vi "_047.vi"() -> ()   [LabVIEW 2024]
panel:
  out "appended array":dbl[](array[numeric])
  out "initialized array 2":dbl[][](array[numeric])
  out "initialized array":dbl[](array[numeric])
  out "Array 4":i32[][](array[numeric])
  out "Array 3":i32[](array[numeric])
  in  "Array":dbl[](array[numeric])
  in  "Array":dbl[](array[numeric])
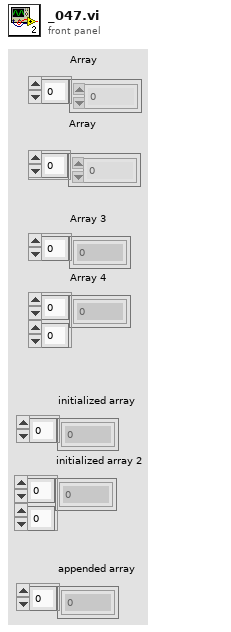
[diagram p1: front panel]
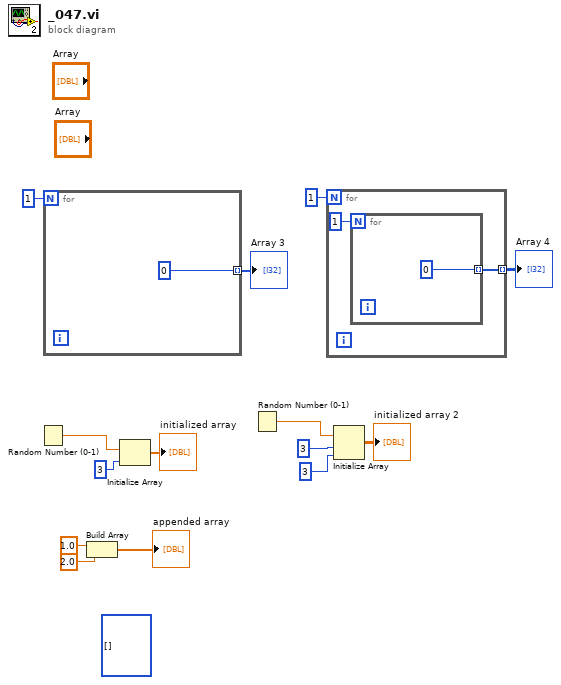
[diagram p0: block diagram]
diagram:
  (unwired) i32[] []
  n1 = Random Number (0-1)() -> (number: 0 to 1=w12:dbl)
  n2 = for {
    N: 1 -> [_]
    tunnel: [0] -> w14 mode=indexing
  }
  "Array 3" <- w14
  n3 = Build Array "Build Array"(1.0 ("element"), 2.0 ("element")) -> (→"appended array":dbl[])
  n4 = Initialize Array(w12, 3) -> (→"initialized array":dbl[])
  n5 = Random Number (0-1)() -> (number: 0 to 1=w8:dbl)
  n6 = for {
    N: 1 -> [_]
    tunnel: [w17] -> w13 mode=indexing
    n7 = for {
      N: 1 -> [_]
      tunnel: [0] -> w17 mode=indexing
    }
  }
  "Array 4" <- w13
  n8 = Initialize Array(w8, 3, 3) -> (→"initialized array 2":dbl[][])
